vi "LED Settings.vi"() -> ()   [LabVIEW 2026]
panel:
  out "appended array":bool[](array[boolean])=[TRUE, FALSE, FALSE, FALSE, FALSE, FALSE, FALSE, FALSE, FALSE, FALSE, FALSE, FALSE, FALSE, FALSE, FALSE, FALSE, FALSE, FALSE, FALSE, FALSE, TRUE, TRUE, TRUE, TRUE, TRUE, FALSE, FALSE, FALSE, TRUE, FALSE, FALSE, FALSE, FALSE, FALSE, FALSE, FALSE, FALSE, FALSE, FALSE, FALSE, FALSE, FALSE, FALSE, FALSE, FALSE]
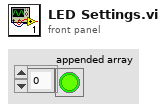
[diagram p1: front panel]
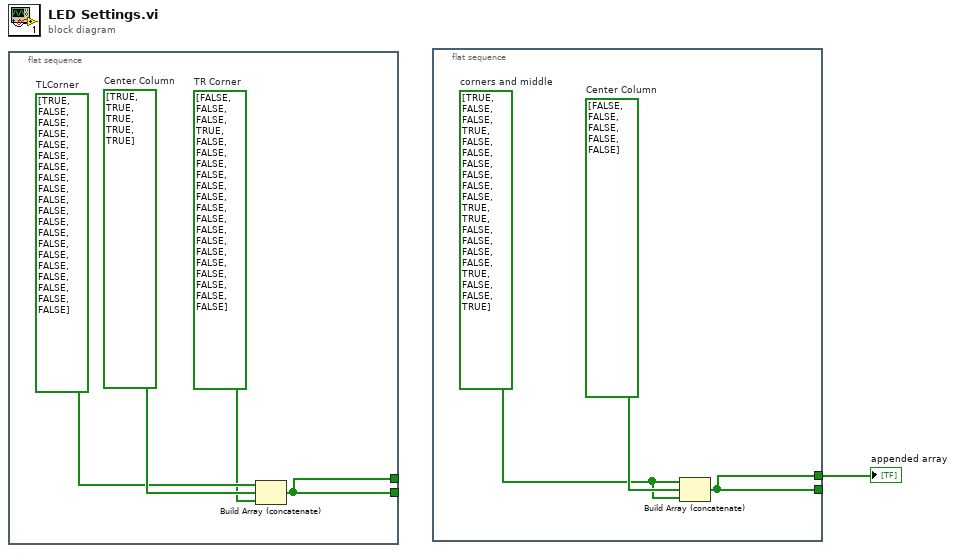
[diagram p0: block diagram]
diagram:
  n1 = flat-sequence {
    tunnel: [w2] -> _
    tunnel: [w2] -> _
    frame #0 {
      w3 = bool[] [FALSE, FALSE, FALSE, TRUE, FALSE, FALSE, FALSE, FALSE, FALSE, FALSE, FALSE, FALSE, FALSE, FALSE, FALSE, FALSE, FALSE, FALSE, FALSE, FALSE]  # TR Corner
      w5 = bool[] [TRUE, TRUE, TRUE, TRUE, TRUE]  # Center Column
      w4 = bool[] [TRUE, FALSE, FALSE, FALSE, FALSE, FALSE, FALSE, FALSE, FALSE, FALSE, FALSE, FALSE, FALSE, FALSE, FALSE, FALSE, FALSE, FALSE, FALSE, FALSE]  # TLCorner
      n2 = Build Array (concatenate)(w4, w5, w3) -> (w2:bool[])
    }
  }
  n3 = flat-sequence {
    tunnel: [w7] -> _
    tunnel: [w7] -> w1
    frame #0 {
      w8 = bool[] [FALSE, FALSE, FALSE, FALSE, FALSE]  # Center Column
      w6 = bool[] [TRUE, FALSE, FALSE, TRUE, FALSE, FALSE, FALSE, FALSE, FALSE, FALSE, TRUE, TRUE, FALSE, FALSE, FALSE, FALSE, TRUE, FALSE, FALSE, TRUE]  # corners and middle
      n4 = Build Array (concatenate)(w6, w8, w6) -> (w7:bool[])
    }
  }
  "appended array" <- w1
